vi "emi_Global Seconds since First Call.vi"(11 "error in (no error)":errorcluster) -> (8 "Seconds since Program Start":u32, 15 "error out":errorcluster)   [LabVIEW 2010]
doc: "Returns number of secounds(time format) since first time called. Global, for determening application uptime.\nOn Error In: No change\n\nSubroutine"
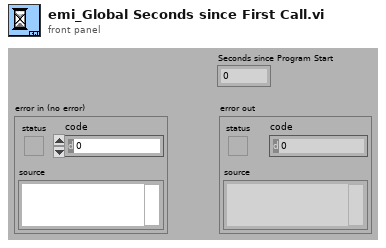
[diagram p1: front panel]
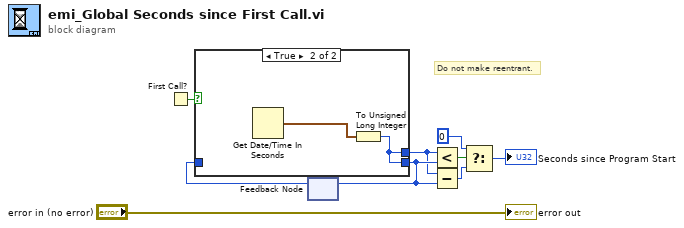
[diagram p0: block diagram]
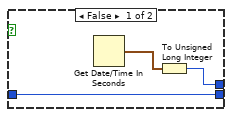
[diagram p2: hidden frame]
diagram:
  # "Do not make reentrant."
  n1 = First Call?() -> (First Call?: T/F=w2:bool)
  n2 = feedback #1() -> (w3:u32)  [unwired: 1 in]
  n3 = case shown="True" w2 {
    tunnel: [w11 w14] -> w7
    tunnel: w3 -> [w11 _]
    tunnel: [w12 w14] -> w6
    frame False {
      n4 = Get Date/Time In Seconds() -> (seconds since 1Jan1904=w10:timestamp)
      n5 = To Unsigned Long Integer(number=w10) -> (unsigned 32bit integer=w12:u32)
    }
    frame True {
      n6 = Get Date/Time In Seconds() -> (seconds since 1Jan1904=w13:timestamp)
      n7 = To Unsigned Long Integer(number=w13) -> (unsigned 32bit integer=w14:u32)
    }
  }
  n8 = feedback-in #1(w7) -> ()
  n9 = Less?(x=w6, y=w7) -> (x < y?=w4:bool)
  n10 = Subtract(x=w6, y=w7) -> (x-y=w8:u32)
  n11 = Select(t=u32 0, s=w4, f=w8) -> (s? t:f=→"Seconds since Program Start":u32)
  "error out" <- "error in (no error)"
